vi "FTW-Package-Initialize.vi"(0 "FTW Message":refnum<class "FTW-Package.lvclass">, 5 "Sender Identity":string, 7 "Message Header":string, 9 "Message Body":string, 11 "error in":errorcluster) -> (4 "FTW Message out":refnum<class "FTW-Package.lvclass">, 15 "error out":errorcluster)   [LabVIEW 2013, in "FTW-Package.lvclass"]
uses:
  FTW-Package.lvclass
panel:
  # "Inputs"
  # "Outputs"
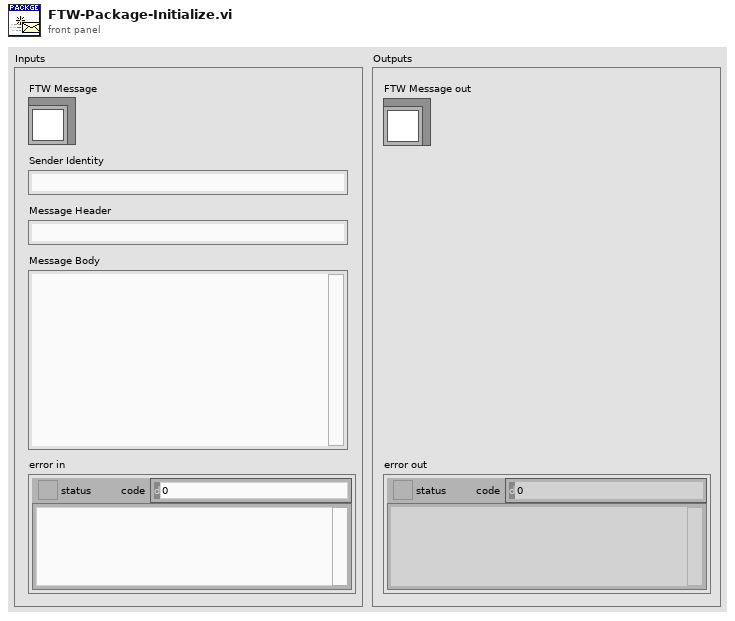
[diagram p1: front panel]
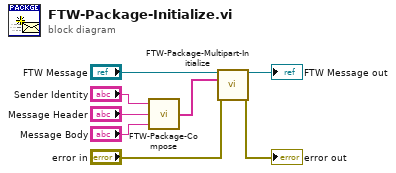
[diagram p0: block diagram]
diagram:
  n1 = call "FTW-Package-Compose.vi"("Message Body"="Message Body", "Message Header"="Message Header", "Sender Identity"="Sender Identity") -> ("Multipart Message"=w3:string[])  [unwired: 1 in]
  n2 = call-dynamic "FTW-Package-Multipart-Initialize.vi"("FTW Message"="FTW Message", "Message Parts"=w3, "error in"="error in") -> ("FTW Message out"=→"FTW Message out":refnum<class "FTW-Package.lvclass">, "error out"=→"error out":errorcluster)  [unwired: 11 in]
